vi "Copy Memory Address to Image (Greyscale).vi"(8 "error in (no error)":errorcluster, 10 "Greyscale Destination Image":T1, 11 "Source":T2) -> (0 "error out":errorcluster, 3 "Greyscale Destination Image (duplicate)":T1)   [LabVIEW 2020, in "g_ar_toolkit.image.lvlib"]
uses:
  g_ar_toolkit.image.lvlib
  Raw Memory Information.ctl
  Raw Memory Information Dimension.ctl
  Greyscale Image.ctl
  e0109ec8-11ee-4a07-aeee-d632e4e22c38.vi
  g_ar_toolkit.common/Module Path.vi
  <vilib>/Utility/error.llb/Error Cluster From Error Code.vi
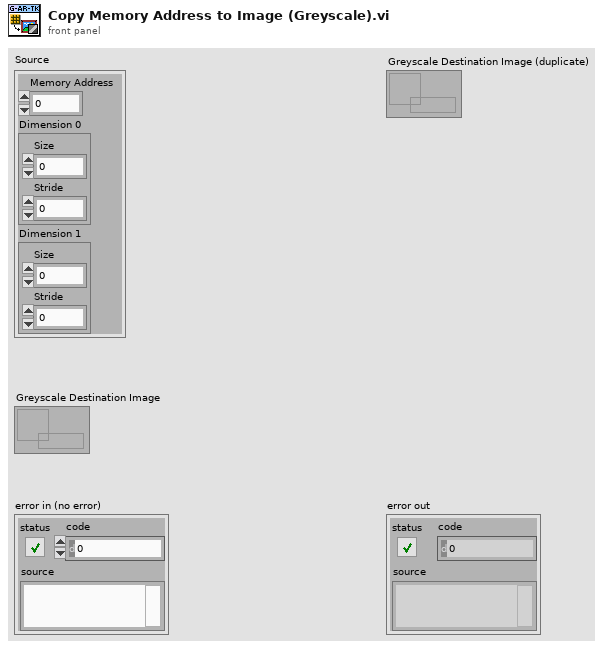
[diagram p1: front panel]
types:
  T1 = typedef "g_ar_toolkit.image.lvlib/Greyscale Image.ctl" = refnum<data-value>
  T2 = typedef "g_ar_toolkit.image.lvlib/Raw Memory Information.ctl" = cluster{"Memory Address":u64, "Dimension 0":T3, "Dimension 1":T3}
  T3 = typedef "g_ar_toolkit.image.lvlib/Raw Memory Information Dimension.ctl" = cluster{"Size":u16, "Stride":u32}
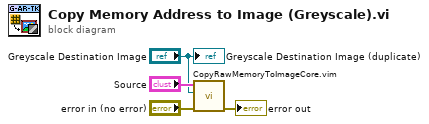
[diagram p0: block diagram]
diagram:
  n1 = call "CopyRawMemoryToImageCore.vim"("error in (no error)"="error in (no error)", "Dst"="Greyscale Destination Image", "Source"="Source") -> ("error out"=→"error out":errorcluster)  [unwired: 8 in]
  "Greyscale Destination Image (duplicate)" <- "Greyscale Destination Image"
